vi "Actor Core.vi"(8 "error in":errorcluster, 11 "Analog Input Channel in":refnum<class "Analog Input Channel.lvclass">) -> (0 "error out":errorcluster, 3 "Actor out":refnum<class "Actor.lvclass">)   [LabVIEW 2015, in "Analog Input Channel.lvlib" / "Analog Input Channel.lvclass"]
doc: "(<B>Filename</B>: Actor Framework.lvlib:Actor.lvclass:Actor Core.vi)\n\nReceives messages to the actor, reacts to them, and initiates any error handling that may shut the actor down.\n\nDescendant classes may override this VI to append parallel tasks for the actor to complete while it handles messages. Overrides use the Call Parent Method node."
uses:
  Analog Input Channel.lvclass
  <vilib>/ActorFramework/Actor/Actor.lvclass
  Input Channel/Input Channel/Input Channel.lvclass
  <userlib>/_Win8uiFramework/ViewableActor.lvclass
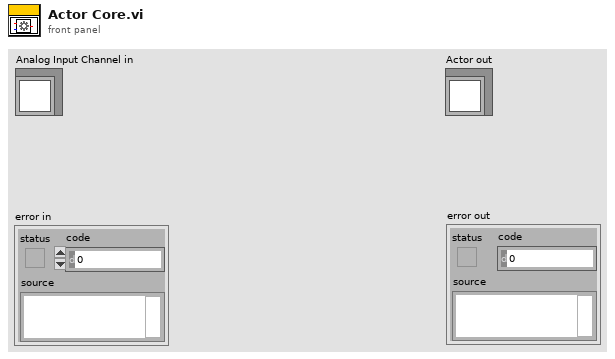
[diagram p1: front panel]
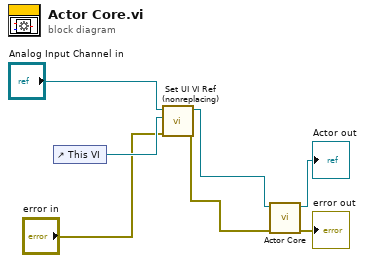
[diagram p0: block diagram]
diagram:
  n1 = control-ref of="This VI"() -> (w5:refnum<vi>)
  n2 = call <userlib>:"Set UI VI Ref (nonreplacing).vi"("error in (no error)"="error in", "UI VI Ref"=w5, "ViewableActor in"="Analog Input Channel in") -> ("error out"=w1:errorcluster, "ViewableActor out"=w3:refnum<class "Analog Input Channel.lvclass">)  [unwired: 6 in, 1 out]
  n3 = call-parent "Actor Core.vi"("error in"=w1, "Channel in"=w3) -> ("error out"=→"error out":errorcluster, "Actor out"=→"Actor out":refnum<class "Actor.lvclass">)  [unwired: 8 in]
